vi "Main.vi"() -> ()   [LabVIEW 2013] (continued)
            n812 = call "DB - [Setup].[Item] (Part Details).vi"("DB - Setup Item Enum"=DB_-_Setup_Item_Enum."SELECT [Setup].[ProcedureItem]", "DB.Schema.Table Array"=w1315, "Transaction"=w1292, "DB Refnums"=w1314) -> ("SUMMARY"=w1293:errorcluster)  [unwired: 6 in, 5 out]
            n813 = control-ref of="MCListBox FHS Setup"() -> (w1304:refnum<vi>)
            n814 = local read "WPS Details Setup"() -> (w1310:T8)
            n815 = call "ET3500 - Write Program.vi"("Simulate"=w1309, "Error In"=w1293, "MCListBox FHS Setup"=w1304, "WPS Details Setup"=w1310) -> ("Final Target Temperture"=w1306:i32, "Seq-Seg Info"=w1305:T17)  [unwired: 2 in, 4 out]
            n816 = Number To Decimal String(number=w1306) -> (decimal integer string=w1307:string)  [unwired: 1 in]
            n817 = local write "Seq-Seg Info"(w1305) -> ()
            n818 = Bundle(w1307) -> (w1308:cluster{string})  [unwired: 1 in]
            n819 = local write "Final Target Temperature"(w1308) -> ()
            n820 = Unbundle By Name(w1292) -> ("[TransactionNo]"=w1299:string, "[TransactionRunNo]"=w1303:string)
            n821 = Empty String/Path?(string/path=w1303) -> (empty?=w1298:bool)
            n822 = Select(t="", s=w1298, f=", ") -> (s? t:f=w1302:string)
            n823 = Concatenate Strings(w1299, w1302, w1303) -> (w1297:string)
            n824 = case shown="Error" w1293 {
              tunnel: ["<I 219>" ("<.?....> Message Code") "<E 218>" ("<.?....> Message Code")] -> w1294
              tunnel: ["Transaction Loaded Successfully" ("Short Description (When DB Not Available)") "Transaction Load Fail" ("Short Description (When DB Not Available)")] -> w1295
              tunnel: [" details loaded." ("Description (When DB Not Available)") " cannot be loaded." ("Description (When DB Not Available)")] -> w1296
              frame No Error {
              }
              frame Error {
              }
            }
            n825 = call "Msgbox - Message Handler.vi"("Short Description (When DB Not Available)"=w1295, "Description (When DB Not Available)"=w1296, "Pre-Description"=w1297, "<.?....> Message Code"=w1294) -> ("MHandler Error"=w1291:errorcluster)  [unwired: 5 in, 2 out]
            n826 = local write "MHandler"(w1291) -> ()
          }
          frame True {
            # "Msgbox - Message Handler is already inside"
            # "Event Fired from Search Button"
            n827 = local write "From Search Button"(FALSE ("From Search Button")) -> ()
            n828 = call "DB UI - Search-Load Setup.vi"("Refnums"=w1336) -> ("Error Out"=w1332:errorcluster, "{Cancel}"=w1334:bool, "Transaction"=w1338:T19)  [unwired: 7 in, 1 out]
            n829 = Not(x=w1334) -> (.not. x?=w1333:bool)
            n830 = local write "MHandler"(w1332) -> ()
            n831 = case shown="False" w1333 {
              tunnel: w1338 -> [_ w1341]
              tunnel: [_ w1341] -> w1335
              frame False {
                # "CANCEL is Clicked"
                n832 = call "Queue - EnQueue to MessageQ.vi"("<NoD> Don't Display to UI"=TRUE, "Message"="{Search Setup} Cancelled by user. ") -> ()  [unwired: 9 in, 1 out]
              }
              frame True {
                # "CANCEL NOT Clicked"
                n833 = Unbundle By Name(w1341) -> ("TransactionNo"=w1343:string, "TransactionRunNo"=w1342:string)
                n834 = global write "Global SRTRS.vi" "[TransactionRunNo]"(w1342) -> ()
                n835 = global write "Global SRTRS.vi" "[TransactionNo]"(w1343) -> ()
              }
            }
          }
        }
        n836 = case shown="True" w1250 {
          tunnel: w1253 -> [_ w1290]
          frame False {
          }
          frame True {
            w1271 = string[] ["TC1", "TC2", "TC3", "TC4", "TC5", "TC6"]  # Channel to Probe Cluster Label
            # "Set to NEXT blank value"
            # "Temperature and Time Variant NOT written here."
            # "Do we want to update these values during Load Setup?"
            n837 = control-ref of="Part Details"() -> (w1264:refnum<vi>)
            n838 = control-ref of="WPS Details Setup"() -> (w1263:refnum<vi>)
            n839 = control-ref of="Extra WPS"() -> (w1255:refnum<vi>)
            n840 = property class="Clust (strict)"(reference=w1263) -> ("Value"=w1285:T8)  [unwired: 1 in, 2 out]
            n841 = property class="Str"(reference=w1255) -> ("Value"=w1254:string)  [unwired: 1 in, 2 out]
            n842 = Unbundle By Name(w1290) -> ("TransactionRunNo"=w1268:string)
            n843 = property class="MCListbox (strict)"(reference=w1264) -> (reference out=w1257:refnum<vi>, "ColHdrString"=w1276:string[], "ItemNames"=w1277:string[][])  [unwired: 1 in, 1 out]
            n844 = control-ref of="MCListBox FHS Setup"() -> (w1265:refnum<vi>)
            n845 = local read "Edit WPS in Setup"() -> (w1269:bool)
            n846 = control-ref of="Tab Setup"() -> (w1287:refnum<vi>)
            n847 = control-ref of="No."() -> (w1261:refnum<vi>)
            n848 = Unbundle By Name(w1285) -> ("WPS/Ref"=w1281:T5, "WPS Details Temperature Units"=w1282:string, "Hold Temperature"=w1283:string, "Hold Time (HH:MM)"=w1284:string)
            n849 = Equal?(x=w1268, y="") -> (x = y?=w1266:bool)
            n850 = call "Setup Tab - Enable-Disable.vi"("No."=w1261, "MCListBox FHS Setup"=w1265, "[SRTRS][Config][ParameterSettings] - [userEditableProcedure]"=w1269, "Disabled"=T30."Disabled", "Tab Setup"=w1287) -> ()  [unwired: 7 in]
            n851 = local read "Channel to Probe Mapping"() -> (w1270:cluster{"Channel to Probe Mapping":string})
            n852 = Unbundle By Name(w1270) -> ("Channel to Probe Mapping"=w1272:string)
            n853 = local write "Uploaded to ET"(FALSE ("Uploaded to ET")) -> ()
            n854 = Not(x=w1266) -> (.not. x?=w1259:bool)
            n855 = Array Size(array=w1277) -> (size(s)=w1278:i32[])
            n856 = Index Array(array=w1278) -> (element=w1256:i32)  [unwired: 1 in]
            n857 = property on="TransactionRunNo" class="Str"("Visible"=w1259) -> ()  [unwired: 2 in, 2 out]
            n858 = call "String - Channel to Probe Mappings.vi"("Channel to Probe Mapping"=w1272, "Channel to Probe Cluster Label"=w1271, "ColHdrString"=w1276, "ItemNames"=w1277) -> ("Probe List Valid"=w1274:bool, "Probe List"=w1273:i32[], "cRIO Channel List"=w1275:i32[])  [unwired: 1 in, 4 out]
            n859 = local write "Probe List Valid"(w1274) -> ()
            n860 = local write "Probe List"(w1273) -> ()
            n861 = local write "cRIO Channel List"(w1275) -> ()
            n862 = local write "No. of Items"(w1256) -> ()
            n863 = property on="Transaction Details" class="Bool"("Visible"=w1259) -> ()  [unwired: 2 in, 2 out]
            n864 = local read "Info."() -> (w1279:T9)
            n865 = Bundle By Name(cluster=w1279, "Ref WPS"=w1281, "WPS"=w1254, "Info. Temperature Units"=w1282, "Info. Temperature Units 2"=w1282, "Hold. Temp."=w1283, "Hold. Time (hour:minute)"=w1284) -> (w1280:T9)
            n866 = local write "Info."(w1280) -> ()
            n867 = Increment(x=w1256) -> (x+1=w1258:i32)
            n868 = property class="MCListbox (strict)"(reference=w1257, "Val(Sgnl)"=w1256) -> ()  [unwired: 1 in, 2 out]
            n869 = property on="Setup Edit" class="Bool (strict)"("Value"=FALSE ("Setup Edit")) -> ()  [unwired: 2 in, 2 out]
            n870 = property on="No." class="DigNum (strict)"("Value"=w1258) -> ()  [unwired: 2 in, 2 out]
            n871 = Unbundle By Name(w1290) -> ("TransactionNo"=w1289:string, "TransactionRunNo"=w1288:string)
            n872 = local write "TransactionRunNo (Execute)"(w1288) -> ()
            n873 = local write "Transaction No (Execute)"(w1289) -> ()
            n874 = global write "Global SRTRS.vi" "[TransactionRunNo]"(w1288) -> ()
            n875 = global write "Global SRTRS.vi" "[TransactionNo]"(w1289) -> ()
            n876 = local write "TransactionRunNo"(w1288) -> ()
            n877 = local write "Transaction No"(w1289) -> ()
          }
        }
      }
      event "Transaction Details": Value Change {
        n878 = event-data() -> ()  [unwired: 1 in, 6 out]
        n879 = local read "Transaction No"() -> (w1347:string)
        n880 = local read "TransactionRunNo"() -> (w1346:string)
        n881 = Bundle("Transaction No"=w1347, "TransactionRunNo"=w1346) -> (w1345:T61)  [unwired: 1 in]
        n882 = call "DB UI - Transaction Details.vi"("Transaction"=w1345) -> ("SUMMARY"=w1344:errorcluster)  [unwired: 9 in, 1 out]
        n883 = local write "DB"(w1344) -> ()
      }
      event "SAPProduction Long Text": Value Change {
        n884 = event-data() -> ()  [unwired: 1 in, 6 out]
        n885 = property on="Order No." class="Str"() -> ("Value"=w1350:string)  [unwired: 2 in, 2 out]
        n886 = local read "Logon"() -> (w1349:T21)
        n887 = Unbundle By Name(w1349) -> ("PlantID"=w1348:string)
        n888 = call "DB UI - MasterData SAPProduction Long Text.vi"("[OrderNo]"=w1350, "[PlantId]"=w1348) -> ()  [unwired: 8 in, 2 out]
      }
      event "SAPMaterial Description (Long) Setup Tab", "SAPMaterial Description (Long) Master Data Tab": Value Change {
        n889 = event-data() -> ("CtlRef"=w1353:refnum<vi>)  [unwired: 1 in, 5 out]
        n890 = property class="Bool"(reference=w1353) -> ("Label.Text"=w1352:string)  [unwired: 1 in, 2 out]
        n891 = case shown="\"SAPMaterial Description (Long) Master Data Tab\", Default" w1352 {
          tunnel: [w1357 w1358] -> w1351
          frame "SAPMaterial Description (Long) Master Data Tab", Default {
            n892 = property on="Master Data Material" class="CmbBox"() -> ("Value"=w1357:string)  [unwired: 2 in, 2 out]
          }
          frame "SAPMaterial Description (Long) Setup Tab" {
            n893 = property on="Material" class="CmbBox"() -> ("Value"=w1358:string)  [unwired: 2 in, 2 out]
          }
        }
        n894 = local read "Logon"() -> (w1356:T21)
        n895 = Unbundle By Name(w1356) -> ("LanguageID"=w1355:string)
        n896 = call "DB UI - MasterData SAPMaterial (Long) Description.vi"("FP is Modal"=TRUE ("UI Popup"), "[LanguageId]"=w1355, "[MaterialNo]"=w1351) -> ()  [unwired: 6 in, 3 out]
      }
      event "Read ET3500 Program": Value Change {
        n897 = event-data() -> ()  [unwired: 1 in, 6 out]
        n898 = local read "VISA resource name RS232"() -> (w1362:string)
        n899 = local read "Simulate ET3500"() -> (w1359:bool)
        n900 = call "ET3500 - Read Program.vi"("subVI"=TRUE, "Simulate"=w1359, "VISA resource name"=w1362) -> ("error out"=w1360:errorcluster)  [unwired: 6 in, 2 out]
        n901 = local write "ET3500 Error"(w1360) -> ()
      }
      event "cRIO Set Time": Value Change {
        n902 = event-data() -> ()  [unwired: 1 in, 6 out]
        n903 = call "Password to adjust CompactRIO internal Clock"() -> ("Password"=w1367:string, "OK"=w1368:bool)  [unwired: 17 in, 1 out]
        n904 = case shown="True" w1368 {
          tunnel: w1367 -> [_ w1371]
          tunnel: ["Cancelled.\n" ("message") w1370] -> w1366
          frame False {
          }
          frame True {
            n905 = case shown="\"3504\"" w1371 {
              tunnel: [w1372 "Password OK.\n"] -> w1370
              frame "False", Default {
                w1372 = "Wrong Password.\n" ("message")
                n906 = One Button Dialog(message=w1372) -> ()  [unwired: 1 in, 1 out]
              }
              frame "3504" {
                n907 = local read "Simulate cRIO"() -> (w1375:bool)
                n908 = case shown="False" w1375 {
                  selector: w1375 -> [w1378 _]
                  tunnel: [w1377 _] -> w1373
                  frame False {
                    # "If we are using \"time zone\" string:\nTime Zone strings need to be of the form Etc/GMT-X or Etc/GMT+X where X represents the offset from GMT. For example Etc\\GMT-6 is the equivalent to Central Standard Time in the US. (GMT-5 during Daylight Saving Time). Valid values range from 12 to -13 centered around GMT."
                    n909 = Get Date/Time In Seconds() -> (seconds since 1Jan1904=w1382:timestamp)
                    n910 = case shown="False" FALSE {
                      tunnel: w1382 -> [w1405 w1407]
                      tunnel: [w1405 w1406] -> w1381
                      frame False {
                      }
                      frame True {
                        # "UTC-7 hours"
                        n911 = Multiply(x=60, y=60) -> (x*y=w1410:i32)
                        n912 = Multiply(x=w1410, y=7) -> (x*y=w1408:i32)
                        n913 = Subtract(x=w1407, y=w1408) -> (x-y=w1406:timestamp)
                      }
                    }
                    n914 = local read "cRIO IP"() -> (w1383:string)
                    n915 = call <vilib>:"Initialize Session.vi"("connect timeout in ms (4s)"=u32 5000, "force property refresh (T)"=TRUE, "target (localhost)"=w1383) -> ("error out"=w1387:errorcluster, "session out"=w1388:refnum<k21>)  [unwired: 7 in]
                    n916 = call <vilib>:"Set Time.vi"("error in (no error)"=w1387, "time"=w1381, "session in (localhost)"=w1388) -> ("error out"=w1386:errorcluster, "session out"=w1389:refnum<k21>)  [unwired: 5 in, 2 out]
                    n917 = call-poly <vilib>:"Close.vi"("error in (no error)"=w1386, "session in"=w1389) -> ("error out"=w1379:errorcluster)  [unwired: 9 in]
                    n918 = flat-sequence {
                      tunnel: w1379 -> [w1390]
                      tunnel: w1378 -> [w1398]
                      tunnel: [w1397] -> w1376
                      tunnel: [w1404] -> w1377
                      tunnel: w1376 -> [w1404]
                      frame #0 {
                        n919 = call "Msgbox - Add OR Remove.vi"("Error In"=w1390, "MsgBox"=T44 {"Show"=TRUE, "Priority"=0, "Message"="Setting cRIO Clock...(Done)", "seconds"=1200}) -> ()  [unwired: 8 in, 2 out]
                      }
                      frame #1 {
                        n920 = local read "cRIO Time Sync Tolerance"() -> (w1392:i32)
                        n921 = local read "cRIO shared variable RT Library"() -> (w1396:string)
                        n922 = Concatenate Strings(w1396, "/cRIO Timestamp" ("cRIO Timestamp SV")) -> (w1394:string)
                        n923 = call "cRIO - Check Time Sync.vi"("Time Sync Tolerance (60sec)"=w1392, "Timeout (minutes)"=2, "cRIO Timestamp SV"=w1394) -> ("error out 4"=w1399:errorcluster)  [unwired: 5 in, 3 out]
                        n924 = local read "cRIO Data Retention"() -> (w1402:i32)
                        n925 = control-ref of="cRIO Status"() -> (w1400:refnum<vi>)
                        n926 = call "cRIO - Shared Variable RW.vi"("shared variable RT Library"=w1396, "Read/Write"=cRIO_RW_Enum."Write Others", "Error In"=w1399, "Simulate cRIO"=w1398, "cRIO Data Retention"=w1402, "cRIO Status"=w1400) -> ("Error Out"=w1397:errorcluster)  [unwired: 5 in, 8 out]
                      }
                      frame #2 {
                        n927 = call "Msgbox - Add OR Remove.vi"("MsgBox"=T44 {"Show"=FALSE, "Priority"=0, "Message"="Setting cRIO Clock...(Done)", "seconds"=1200}) -> ()  [unwired: 9 in, 2 out]
                      }
                    }
                  }
                  frame True {
                    n928 = One Button Dialog(message="cRIO Simulate Set Time OK.") -> ()  [unwired: 1 in, 1 out]
                  }
                }
                n929 = local write "cRIO Error"(w1373) -> ()
              }
            }
          }
        }
        n930 = Concatenate Strings("[cRIO Set Time] Clicked by User. " ("element"), w1366) -> (w1364:string)
        n931 = call "Queue - EnQueue to MessageQ.vi"("<NoD> Don't Display to UI"=TRUE, "Message"=w1364) -> ()  [unwired: 9 in, 1 out]
      }
      event Mouse Down? {
        n932 = event-data() -> ()  [unwired: 1 in, 8 out]
        n933 = local read "DB - Master Data Load"() -> (w1414:bool)
        n934 = case shown="True" w1414 {
          frame False {
          }
          frame True {
            n935 = global read "Global SRTRS.vi" "Logon"() -> (w1419:T21)
            n936 = Unbundle By Name(w1419) -> ("PlantID"=w1418:string)
            n937 = call "DB - [MasterData].[OutputSet].vi"("[PlantId]"=w1418) -> ("2D data"=w1417:string[][])  [unwired: 6 in, 4 out]
            "[OutputSetId],[Description]" <- w1417
            n938 = Index Array(array=w1417, index (col)=0 ("disabled index (col)")) -> (element=w1415:string[])  [unwired: 1 in]
            n939 = property on="Output Set" class="CmbBox (strict)"("Strings[]"=w1415) -> ()  [unwired: 2 in, 2 out]
          }
        }
        n940 = event-data() -> ()  [unwired: 2 in, 1 out]
      }
      event Value Change {
        # "Set [Description] based on [OutputSetId] Chosen"
        # "Set [Description] based on [OutputSetId] Chosen"
        n941 = event-data() -> ("NewVal"=w1424:T5)  [unwired: 1 in, 5 out]
        n942 = local read "[OutputSetId],[Description]"() -> (w1427:string[][])
        n943 = Index Array(array=w1427, index (col) #1=0 ("disabled index (col)"), index (col) #2=1 ("index (col)")) -> (element #1=w1425:string[], element #2=w1421:string[])  [unwired: 2 in]
        n944 = Search 1D Array(1D array=w1425, element=w1424) -> (index of element=w1423:i32)  [unwired: 1 in]
        n945 = Index Array(array=w1421, index=w1423) -> (element=w1420:string)
        n946 = property on="Description" class="Str"("Value"=w1420) -> ()  [unwired: 2 in, 2 out]
      }
      event "Setup Load Debug": Value Change {
        w1455 = string[] ["TC1", "TC2", "TC3", "TC4", "TC5", "TC6"]  # Channel to Probe Cluster Label
        # "We are using CellBG Unused Cells color for both\nMCListBox FHS Setup\nMCListBox AWPS"
        # "Part Details\nMCListBox FHS Setup\nMCListBox AWPS"
        # "Only WPS Detais Setup"
        # "MCListBox FHS Setup\nMCListBox AWPS"
        # "For Debug ONLY"
        n947 = event-data() -> ()  [unwired: 1 in, 6 out]
        n948 = control-ref of="WPS Details Setup"() -> (w1438:refnum<vi>)
        n949 = Index Array(array=w1463, index #1=0 ("index"), index #2=1 ("index"), index #3=2 ("index")) -> (element #1=w1450:refnum<vi>, element #2=w1462:refnum<vi>, element #3=w1461:refnum<vi>)
        n950 = local read "Setup"() -> (w1434:path)
        n951 = Build Array(w1450, w1462, w1461) -> (w1460:refnum<vi>[])
        n952 = Format Date/Time String(time format string (%c)="%Y\\%m") -> (date/time string=w1433:string)  [unwired: 2 in]
        n953 = Build Array "Part Details\nClusters"(w1438) -> (w1464:refnum<vi>[])
        n954 = local read "Channel to Probe Mapping"() -> (w1456:cluster{"Channel to Probe Mapping":string})
        n955 = Unbundle By Name(w1456) -> ("Channel to Probe Mapping"=w1454:string)
        n956 = Build Path(base path=w1434, name or relative path=w1433) -> (appended path=w1432:path)
        n957 = call "File Dialog"("start path"=w1432, "prompt"="Select SETUP file", "pattern (all files)"="*.stp" ("pattern label")) -> ("selected path"=w1476:path, "error out"=w1480:errorcluster)  [unwired: 9 in, 2 out]
        n958 = call <vilib>:"Open Config Data.vi"("error in (no error)"=w1480, "configuration file path"=w1476) -> ("error out"=w1479:errorcluster, "refnum"=w1481:T59)  [unwired: 7 in, 1 out]
        n959 = Strip Path(path=w1476) -> (name=w1475:string)  [unwired: 1 out]
        n960 = for {
          tunnel: w1460 -> [w1495] mode=indexing
          tunnel: w1481 -> [w1499]
          tunnel: w1479 -> [w1498]
          tunnel: [w1497] -> w1478
          tunnel: [w1496] -> w1477
          n961 = call "Key - MCListbox Read.vi"("error in (no error)"=w1498, "New MulticolumnListbox Ref"=w1495, "Original MulticolumnListbox Ref"=w1495, "refnum"=w1499) -> ("error out"=w1496:errorcluster, "Refnum out"=w1497:T59)  [unwired: 4 in, 2 out]
        }
        n962 = Match Pattern(string=w1475, regular expression="[_]") -> (before substring=w1430:string)  [unwired: 1 in, 3 out]
        n963 = global write "Global SRTRS.vi" "[TransactionNo]"(w1430) -> ()
        n964 = local write "Transaction No (Execute)"(w1430) -> ()
        n965 = local write "Transaction No"(w1430) -> ()
        n966 = for {
          tunnel: w1464 -> [w1490] mode=indexing
          tunnel: w1478 -> [w1494]
          tunnel: w1477 -> [w1493]
          tunnel: [w1492] -> w1470
          tunnel: [w1491] -> w1471
          n967 = call "Key - Cluster Read.vi"("error in (no error)"=w1493, "New Ctl Ref"=w1490, "Original Ctl Ref"=w1490, "Refnum in"=w1494) -> ("error out"=w1492:errorcluster, "Refnum out"=w1491:T59)  [unwired: 5 in, 1 out]
        }
        n968 = call <vilib>:"Close Config Data.vi"("error in (no error)"=w1470, "refnum"=w1471) -> ("error out"=w1448:errorcluster, "file path"=w1482:path)  [unwired: 8 in]
        n969 = property class="MCListbox (strict)"(reference=w1450, error in=w1448) -> (error out=w1436:errorcluster, "ColHdrString"=w1449:string[], "ItemNames"=w1441:string[][])  [unwired: 1 out]
        n970 = property class="Clust (strict)"(reference=w1438, error in=w1436) -> (error out=→"Property Node Error":errorcluster, "Value"=w1437:T8)  [unwired: 1 out]
        n971 = Array Size(array=w1441) -> (size(s)=w1440:i32[])
        n972 = Unbundle By Name(w1437) -> ("WPS/Ref"=w1445:T5, "WPS Details Temperature Units"=w1444:string, "Hold Temperature"=w1443:string, "Hold Time (HH:MM)"=w1442:string)
        n973 = Index Array(array=w1440) -> (element=w1439:i32)  [unwired: 1 in]
        n974 = call "String - Channel to Probe Mappings.vi"("Channel to Probe Mapping"=w1454, "Channel to Probe Cluster Label"=w1455, "ColHdrString"=w1449, "ItemNames"=w1441) -> ("Probe List Valid"=w1452:bool, "Probe List"=w1453:i32[], "cRIO Channel List"=w1451:i32[])  [unwired: 1 in, 4 out]
        n975 = local write "Probe List Valid"(w1452) -> ()
        n976 = local write "Probe List"(w1453) -> ()
        n977 = local write "cRIO Channel List"(w1451) -> ()
        n978 = local write "No. of Items"(w1439) -> ()
        n979 = Index Array(array=w1463, index #1=1 ("index"), index #2=2 ("index")) -> (element #1=w1467:refnum<vi>, element #2=w1466:refnum<vi>)
        n980 = Build Array(w1467, w1466) -> (w1465:refnum<vi>[])
        n981 = local read "Info."() -> (w1447:T9)
        n982 = Bundle By Name(cluster=w1447, "Ref WPS"=w1445, "Info. Temperature Units"=w1444, "Info. Temperature Units 2"=w1444, "Hold. Temp."=w1443, "Hold. Time (hour:minute)"=w1442) -> (w1446:T9)
        n983 = local write "Info."(w1446) -> ()
        n984 = Not A Number/Path/Refnum?(number/path/refnum=w1482) -> (NaN/Path/Refnum?=w1483:bool)
        n985 = for {
          tunnel: w1465 -> [w1489] mode=indexing
          tunnel: w1448 -> [w1488]
          n986 = local read "CellBG Unused Cells"() -> (w1485:u32)
          n987 = call "MCListbox Refresh.vi"("Which Cells"=T46."Exisiting and Blank Cells", "Error In"=w1488, "color of New Cells"=w1485, "color of Blank cells"=w1485, "MulticolumnListbox in"=w1489) -> ("Error Out"=w1486:errorcluster)  [unwired: 5 in, 1 out]
          n988 = local write "Property Node Error"(w1486) -> ()
        }
        n989 = case "MessageQ" shown="False" w1483 {
          tunnel: w1482 -> [w1506 _]
          tunnel: [w1503 w1507] -> w1429
          tunnel: "{Load Setup}" ("result string") -> [w1501 w1509]
          frame False {
            w1504 = "\"" ("string")
            # "File Load OK"
            n990 = Path To String(path=w1506) -> (string=w1505:string)
            n991 = Concatenate Strings(w1501, " OK. " ("string"), w1504, w1505, w1504, " loaded." ("string")) -> (w1503:string)
          }
          frame True {
            # "File Not Loaded"
            n992 = Concatenate Strings(w1509, " Cancelled.") -> (w1507:string)
          }
        }
        n993 = call "Queue - EnQueue to MessageQ.vi"("<NoD> Don't Display to UI"=TRUE, "Message"=w1429) -> ()  [unwired: 9 in, 1 out]
      }
      event "------------------------------------        Execute TAB      ------------------------------------": Value Change {
        n994 = event-data() -> ()  [unwired: 1 in, 6 out]
      }
      event "Recipe Stop", "Recipe Start": Value Change {
        w1511 = 1  # MCListBox FHS Setup
        # "[BUTTON ACTIONS] are logged into MessageQ"
        n995 = event-data() -> ()  [unwired: 1 in, 6 out]
        n996 = Index Array(array=w1512, index=w1511) -> (element=w1510:refnum<vi>)
        n997 = case shown="True" "Recipe Stop" {
          frame False {
          }
          frame True {
            # "User Click STOP"
            n998 = call "Msgbox - Message Handler.vi"("Short Description (When DB Not Available)"="Process Stop", "Description (When DB Not Available)"="Data Logging in progress. Do you want process to stop?", "<.?....> Message Code"="<W 307>") -> ("MHandler Error"=w1651:errorcluster, "OK Out"=w1650:bool)  [unwired: 6 in, 1 out]
            "Manual Stop" <- w1650
            n999 = local write "MHandler"(w1651) -> ()
            n1000 = local write "Recipe Stop Flag"(w1650) -> ()
            n1001 = Select(t="OK." ("Message"), s=w1650, f="Cancel." ("Message")) -> (s? t:f=w1653:string)
            n1002 = Concatenate Strings("{Recipe Stop} User clicks " ("string"), w1653) -> (w1660:string)
            n1003 = call "Queue - EnQueue to MessageQ.vi"("<NoD> Don't Display to UI"=TRUE, "Message"=w1660) -> ()  [unwired: 9 in, 1 out]
          }
        }
        n1004 = case shown="True" "Recipe Start" {
          selector: "Recipe Start" -> [w1516 _]
          tunnel: [w1516 w1518] -> w1513
          tunnel: w1510 -> [_ w1517]
          frame False {
            (unwired) ""
          }
          frame True {
            n1005 = local read "Uploaded to ET"() -> (w1519:bool)
            n1006 = case shown="False" w1519 {
              selector: w1519 -> [_ w1649]
              tunnel: [w1520 w1649] -> w1518
              tunnel: w1517 -> [w1523 _]
              frame False {
                # "Current [TransactionNo] (and) [TransactionRunNo] may not be the last one UPLOADED to ET. Must UPLOAD again."
                n1007 = local read "VISA resource name RS232"() -> (w1526:string)
                n1008 = local read "WPS Details Setup"() -> (w1527:T8)
                n1009 = local read "Simulate ET3500"() -> (w1525:bool)
                n1010 = call "ET3500 - Write Program.vi"("Simulate"=w1525, "MCListBox FHS Setup"=w1523, "WPS Details Setup"=w1527, "VISA resource name RS232"=w1526) -> ("ET3500"=w1521:errorcluster, "Final Target Temperture"=w1524:i32, "Seq-Seg Info"=w1522:T17)  [unwired: 2 in, 3 out]
                n1011 = local write "Seq-Seg Info"(w1522) -> ()
                n1012 = flat-sequence {
                  tunnel: w1524 -> [w1530]
                  frame #0 {
                    n1013 = Number To Decimal String(number=w1530) -> (decimal integer string=w1529:string)  [unwired: 1 in]
                    n1014 = Bundle(w1529) -> (w1528:cluster{string})  [unwired: 1 in]
                    n1015 = property on="Final Target Temperature" class="Clust (strict)"("Value"=w1528) -> ()  [unwired: 2 in, 2 out]
                  }
                }
                n1016 = local write "ET3500 Error"(w1521) -> ()
                n1017 = case shown="No Error" w1521 {
                  tunnel: w1525 -> [w1532 _]
                  tunnel: [w1531 FALSE] -> w1520
                  frame No Error {
                    n1018 = while {
                      tunnel: w1532 -> [w1536]
                      tunnel: [w1533] -> w1531
                      i -> [w1535]
                      stop <- w1534 stop-if-true
                      n1019 = case shown="2, Default" w1535 {
                        tunnel: w1536 -> [_ _ w1618]
                        tunnel: [w1548 TRUE w1614] -> w1534
                        tunnel: [w1548 FALSE ("OK Out") w1613] -> w1533
                        frame 1 {
                          w1546 = 7  # Cal. Required
                          (unwired) string[] ["Name", "Model", "Serial No.", "Last Cal. Date", "Next Cal. Due Date", "Equipment ID", "Notice Period", "Cal. Required"]  # 2015-01-01 11:16 ColHdr[]
                          w1556 = 5  # Equipment ID
                          w1562 = 6  # Notice Period
                          w1564 = 4  # Next Cal. Due Date
                          # "Temperature Controller follows Furnace date"
                          # "Equipment ID Notice Due List"
                          # "Not Prompted here. Only in Setup"
                          # "If ALL TRUE End Loop, SET\nUploaded to ET to TRUE"
                          # "Same Check done in {Setup Save}"
                          # "60 x 60 x 24 = 86,400 seconds/day"
                          # "2nd Check: Are Equipment Calibration OK?"
                          n1020 = property on="Equipment Details" class="MCListbox (strict)"() -> ("ItemNames"=w1555:string[][])  [unwired: 2 in, 2 out]
                          n1021 = property on="Next Calibration Due Date" class="Str"() -> ("Value"=w1563:string)  [unwired: 2 in, 2 out]
                          n1022 = Array Size(array=w1555) -> (size(s)=w1554:i32[])
                          n1023 = Index Array(array=w1554) -> (element=w1553:i32)  [unwired: 1 in]
                          n1024 = Index Array(array=w1555, index (col) #1=w1564, index (col) #2=w1562, index (col) #3=w1556, index (col) #4=w1546) -> (element #1=w1537:string[], element #2=w1538:string[], element #3=w1543:string[], element #4=w1545:string[])  [unwired: 4 in]
                          n1025 = Greater Than 0?(x=w1553) -> (x > 0?=w1549:bool)
                          n1026 = local write "Equipment Details Complete"(w1549) -> ()
                          n1027 = Build Array (concatenate)(w1563, w1537) -> ()  [unwired: 1 out]
                          n1028 = call "DB - Convert BIT Type.vi"("BIT Type (eg Inactive) (Array)"=w1545) -> ("Boolean (Array)"=w1542:bool[])  [unwired: 2 in, 2 out]
                          n1029 = Get Date/Time In Seconds() -> (seconds since 1Jan1904=w1544:timestamp)
                          n1030 = property on="Output Set" class="CmbBox (strict)"() -> ("Value"=w1552:T5)  [unwired: 2 in, 2 out]
                          n1031 = Empty String/Path?(string/path=w1552) -> (empty?=w1551:bool)
                          n1032 = local read "Date Format (UserDefined)"() -> (w1541:string)
                          n1033 = for {
                            tunnel: w1537 -> [w1579] mode=indexing
                            tunnel: w1544 -> [w1569]
                            tunnel: [w1573] -> w1539 mode=indexing
                            tunnel: w1538 -> [w1583] mode=indexing
                            tunnel: w1543 -> [w1572] mode=indexing
                            tunnel: [w1572] -> _ mode=indexing if=w1580
                            tunnel: w1541 -> [w1578]
                            tunnel: w1542 -> [w1577] mode=indexing
                            tunnel: [w1572] -> w1540 mode=indexing if=w1571
                            # "All FALSE will\nCreate DUE list"
                            # "Next Cal Due Date - Today\n<= Notice Period"
                            n1034 = Not(x=w1577) -> (.not. x?=w1575:bool)
                            n1035 = call "String - Convert UserDefined Date to SQL Date (YYYY-mm-dd).vi"("Date Format (UserDefined)"=w1578, "Date String (UserDefined)"=w1579) -> ("time stamp"=w1570:timestamp)  [unwired: 7 in, 2 out]
                            n1036 = Decimal String To Number(string=w1583) -> (number=w1581:i32)  [unwired: 2 in, 1 out]
                            n1037 = Greater?(x=w1570, y=w1569) -> (0:w1576:bool)
                            n1038 = Or(x=w1576, y=w1575) -> (x .or. y?=w1573:bool)
                            n1039 = Multiply(x=86400.0, y=w1581) -> (x*y=w1567:dbl)
                            n1040 = Subtract(x=w1570, y=w1569) -> (x-y=w1568:dbl)
                            n1041 = Less Or Equal?(x=w1568, y=w1567) -> (x <= y?=w1566:bool)
                            n1042 = Compound Arithmetic op=OR "OR"(invert w1573, invert w1566, w1575) -> (w1574:bool)
                            n1043 = Not(x=w1574) -> (.not. x?=w1580:bool)
                            n1044 = Not(x=w1573) -> (.not. x?=w1571:bool)
                          }
                          n1045 = Not(x=w1551) -> (.not. x?=w1547:bool)
                          n1046 = local write "Output Set Details Complete"(w1547) -> ()
                          n1047 = Array To Spreadsheet String(delimiter (Tab)=",", array=w1540, 3:"" ("format string")) -> (spreadsheet string=w1558:string)
                          n1048 = local write "Calibration Date OK"(w1539) -> ()
                          n1049 = And Array Elements(Boolean array=w1539) -> (logical AND=w1550:bool)
                          n1050 = Search and Replace String(replace all?=TRUE ("replace all? (F)"), input string=w1558, search string="\r\n") -> (result string=w1565:string)  [unwired: 5 in, 3 out]
                          n1051 = local write "All Calibration Date Valid"(w1550) -> ()
                          n1052 = local write "Equipment ID Due List"(w1565) -> ()
                          n1053 = Compound Arithmetic op=AND(w1550, w1549, w1547) -> (w1548:bool)
                        }
                        frame 2, Default {
                          # "One of these is FALSE"
                          # "Prompt Errors of 2nd Check...if any"
                          n1054 = local read "Equipment Details Complete"() -> (w1586:bool)
                          n1055 = local read "Output Set Details Complete"() -> (w1585:bool)
                          n1056 = local read "All Calibration Date Valid"() -> (w1587:bool)
                          n1057 = case shown="True" w1587 {
                            tunnel: ["<E 213>" w1602] -> w1590
                            tunnel: [" calibration validity expired. Save Cancelled." w1601] -> w1591
                            tunnel: ["Calibration Expired" w1600] -> w1592
                            tunnel: [w1595 _] -> w1589
                            tunnel: w1586 -> [_ w1599]
                            tunnel: w1585 -> [_ w1598]
                            frame False {
                              # "Calibration Expired"
                              n1058 = local read "Equipment ID Due List"() -> (w1595:string)
                            }
                            frame True {
                              # "All Calibration Date Valid"
                              n1059 = case shown="True" w1599 {
                                tunnel: ["<E 214>" w1606] -> w1602
                                tunnel: ["Save Cancelled." w1608] -> w1601
                                tunnel: ["Equipment Not Available. " w1607] -> w1600
                                tunnel: w1598 -> [_ w1609]
                                frame False {
                                # "Equipment Not Available"
                                }
                                frame True {
                                # "Equipment Details Complete"
                                n1060 = case shown="False" w1609 {
                                tunnel: ["Please select a valid Output Set to proceed" _] -> w1608
                                tunnel: ["Output Set Not Assigned" _] -> w1607
                                tunnel: ["<E 215>" _] -> w1606
                                frame False {
                                # "Output Set Details Incomplete"
                                }
                                frame True {
                                # "NA becasue all conditions \nare ANDed\nSo at least one would have failed"
                                # "Output Set Details Complete"
                                }
                                }
                                }
                              }
                            }
                          }
                          n1061 = call "Msgbox - Message Handler.vi"("Short Description (When DB Not Available)"=w1592, "Description (When DB Not Available)"=w1591, "Pre-Description"=w1589, "<.?....> Message Code"=w1590) -> ("MHandler Error"=w1588:errorcluster)  [unwired: 5 in, 2 out]
                          n1062 = local write "MHandler"(w1588) -> ()
                        }
                        frame 0 {
                          # "1st Check: Variants Valid?"
                          n1063 = property on="Variant Allowed (Hold Time)" class="DigNum (strict)"() -> ("Value"=w1622:dbl)  [unwired: 2 in, 2 out]
                          n1064 = property on="Variant Allowed (Hold Temp)" class="DigNum (strict)"() -> ("Value"=w1623:dbl)  [unwired: 2 in, 2 out]
                          n1065 = Equal To 0?(x=w1623) -> (x = 0?=w1621:bool)
                          n1066 = Equal To 0?(x=w1622) -> (x = 0?=w1620:bool)
                          n1067 = Or(x=w1621, y=w1620) -> (x .or. y?=w1619:bool)
                          n1068 = case shown="True" w1619 {
                            tunnel: [TRUE ("OK Out") w1635] -> w1613
                            tunnel: ["" w1630] -> w1617
                            frame False {
                            }
                            frame True {
                              # "Either one is ZERO"
                              n1069 = call "Msgbox - Message Handler.vi"("Short Description (When DB Not Available)"="Temperature/Time Allowance Not Set", "Description (When DB Not Available)"="Variance allowed for Hold. Temperature and Holding Time is not set. Do you want to proceed?", "<.?....> Message Code"="<W 302>") -> ("MHandler Error"=w1637:errorcluster, "OK Out"=w1635:bool)  [unwired: 6 in, 1 out]
                              n1070 = local write "MHandler"(w1637) -> ()
                              n1071 = Select(t="OK.", s=w1635, f="Cancel.") -> (s? t:f=w1631:string)
                              n1072 = Concatenate Strings("User Select ", w1631) -> (w1630:string)
                            }
                          }
                          n1073 = Select(t="Simulate Upload to ET3504 OK." ("message"), s=w1618, f="Upload to ET3504 OK." ("message")) -> (s? t:f=w1624:string)
                          n1074 = Concatenate Strings("{Recipe Start} " ("string"), w1624, w1617) -> (w1615:string)
                          n1075 = call "Queue - EnQueue to MessageQ.vi"("<NoD> Don't Display to UI"=TRUE, "Message"=w1615) -> ()  [unwired: 9 in, 1 out]
                          n1076 = Not(x=w1613) -> (.not. x?=w1614:bool)
                        }
                      }
                    }
                  }
                  frame Error {
                    n1077 = call "Msgbox - Message Handler.vi"("Short Description (When DB Not Available)"="Heating Sequence Upload Fail", "Description (When DB Not Available)"="Heating sequence program upload to furnace controller fail. Check the controller and retry", "<.?....> Message Code"="<E 220>") -> ("MHandler Error"=w1644:errorcluster)  [unwired: 6 in, 2 out]
                    n1078 = local write "MHandler"(w1644) -> ()
                    n1079 = call "Queue - EnQueue to MessageQ.vi"("<NoD> Don't Display to UI"=TRUE, "Message"="{Recipe Start} Upload to ET3504 Failed. Check if ET3504 is already Running a Program. Check communication cable to ET3504." ("message")) -> ()  [unwired: 9 in, 1 out]
                  }
                }
                n1080 = local write "Uploaded to ET"(w1520) -> ()
              }
              frame True {
                # "Already Uploaded, can START"
                n1081 = call "Queue - EnQueue to MessageQ.vi"("<NoD> Don't Display to UI"=TRUE, "Message"="{Recipe Start} ET3504 already uploaded by a previous same TransactionNo." ("string")) -> ()  [unwired: 9 in, 1 out]
              }
            }
          }
        }
        n1082 = local write "Recipe Start Flag"(w1513) -> ()
      }
      event "Parameter": Value Change {
        n1083 = event-data() -> ()  [unwired: 1 in, 6 out]
        n1084 = local read "DB - Transaction"() -> (w1664:bool)
        n1085 = case shown="True" w1664 {
          tunnel: [w1665 w1680] -> w1663
          frame False {
            n1086 = local read "Latest stp file"() -> (w1668:path)
            n1087 = control-ref of="Parameter Buffer"() -> (w1672:refnum<vi>)
            n1088 = call <vilib>:"Open Config Data.vi"("create file if necessary (T)"=FALSE, "configuration file path"=w1668) -> ("error out"=w1666:errorcluster, "refnum"=w1669:T59)  [unwired: 7 in, 1 out]
            n1089 = call "Key - Cluster Read.vi"("error in (no error)"=w1666, "New Ctl Ref"=w1672, "Original Ctl Ref"=w1672, "Refnum in"=w1669) -> ("error out"=w1667:errorcluster, "Refnum out"=w1671:T59)  [unwired: 5 in, 1 out]
            n1090 = call <vilib>:"Close Config Data.vi"("error in (no error)"=w1667, "write file if changed (T)"=FALSE, "refnum"=w1671) -> ("error out"=w1665:errorcluster)  [unwired: 7 in, 1 out]
          }
          frame True {
            w1683 = T62[] [enum."[StartHoldTime]", enum."[EndHoldTime]", enum."[StartHoldTemp]", enum."[EndHoldTemp]"] items=["[StartRecordTime]", "[StartRecordTemp]", "[MaxRecordedTemp]", "[MaxRecordedTempTime]", "[MinRecordedTemp]", "[MinRecordedTempTime]", "[EndRecordTemp]", "[EndRecordTime]", "[RecordedMinutes]", "[StartHoldTime]", "[StartHoldTemp]", "[HoldTimeMaxTemp]", "[HoldTimeMaxTempTime]", "[HoldTimeMinTemp]", "[HoldTimeMinTempTime]", "[EndHoldTime]", "[EndHoldTemp]", "[HoldDurationMinutes]", "[TempDiffDuringHold]", "[UnitOfTemperature]", "[PerformedBy]", "[PerformedOn]", "[IsTempWithinTol]", "[IsTimeWithinTol]", "[HoldTimePercentage]", "[ProcessStatus]", "[OverallStatus]", "[SequenceStatus]", "[Parameter1]", "[Parameter2]", "[Parameter3]", "[Parameter4]", "[Parameter5]", "[Parameter6]", "[Parameter7]", "[Parameter8]", "[Parameter9]", "[Parameter10]", "[Parameter11]", "[Parameter12]", "[Result]", "[RawDataFile]", "[RawDataFilePath]", "[RawDataFileName]", "[OutputSetId]", "[SavedBy]", "[SavedOn]", "[Inactive]"] ("[TransactionResult] v02")
            n1091 = local read "TransactionRunNo"() -> (w1685:string)
            n1092 = local read "Transaction No"() -> (w1686:string)
            n1093 = Bundle("Transaction No"=w1686, "TransactionRunNo"=w1685) -> (w1684:T61)  [unwired: 1 in]
            n1094 = call "DB - [Execute].[Transaction].vi"("DB.Schema.Table"="SRTRS.Execute.TransactionResult", "Transaction"=w1684, "DB - Execute Transaction"=DB_-_Execute_Transaction_Enum."SELECT [TransactionResult]", "[TransactionResult] v02"=w1683) -> ("1D Results"=w1674:string[], "SUMMARY"=w1680:errorcluster)  [unwired: 12 in, 2 out]
            n1095 = Index Array(array=w1674, index #1=0 ("index")) -> (element #1=w1679:string, element #2=w1678:string, element #3=w1677:string, element #4=w1676:string)  [unwired: 3 in]
            n1096 = local read "Parameter Buffer"() -> (w1682:T15)
            n1097 = Bundle By Name(cluster=w1682, "Start Holding Time and Date"=w1679, "End Holding Time and Date"=w1678, "Start Holding Temperature"=w1677, "End Holding Temperature"=w1676) -> (w1681:T15)
            n1098 = local write "Parameter Buffer"(w1681) -> ()
          }
        }
        n1099 = case shown="No Error" w1663 {
          frame No Error {
            n1100 = local read "Parameter Buffer"() -> (w1710:T15)
            n1101 = Unbundle By Name(w1710) -> ("Start Holding Time and Date"=w1704:string, "End Holding Time and Date"=w1702:string, "Start Holding Temperature"=w1709:string, "End Holding Temperature"=w1708:string)
            n1102 = property on="Part Details" class="MCListbox (strict)"() -> ("ItemNames"=w1698:string[][])  [unwired: 2 in, 2 out]
            n1103 = for {
              tunnel: w1698 -> [w1714] mode=indexing
              tunnel: [w1712] -> w1697 mode=indexing
              w1713 = 1  # Order No
              n1104 = Index Array(array=w1714, index=w1713) -> (element=w1712:string)
            }
            n1105 = Fract/Exp String To Number(string=w1709) -> (number=w1707:dbl)  [unwired: 3 in, 1 out]
            n1106 = Fract/Exp String To Number(string=w1708) -> (number=w1706:dbl)  [unwired: 3 in, 1 out]
            n1107 = call "String - Convert Str (YYYY-mm-dd HHcMMcSS) to TimeStamp.vi"("YYYY-mm-dd HH:MM:SS (String)"=w1704) -> ("time stamp"=w1703:timestamp)  [unwired: 9 in, 1 out]
            n1108 = call "String - Convert Str (YYYY-mm-dd HHcMMcSS) to TimeStamp.vi"("YYYY-mm-dd HH:MM:SS (String)"=w1702) -> ("time stamp"=w1701:timestamp)  [unwired: 9 in, 1 out]
            n1109 = property on="Variant Allowed (Hold Temp)" class="Bool (strict)"() -> ("Value"=w1705:bool)  [unwired: 2 in, 2 out]
            n1110 = Array To Spreadsheet String(delimiter (Tab)=",", array=w1697, 3:"" ("format string")) -> (spreadsheet string=w1692:string)
            n1111 = local read "Info."() -> (w1711:T9)
            n1112 = Search and Replace String(replace all?=TRUE ("replace all? (F)"), input string=w1692, search string="\r\n") -> (result string=w1691:string)  [unwired: 5 in, 3 out]
            n1113 = call "Parameters - Update.vi"("Parameter (End Dwell Temp)"=w1706, "Variant Allowed (Summarised)"=w1705, "Parameter (Start Dwell Temp)"=w1707, "Parameter (End Dwell Time)"=w1701, "Parameter (Start Dwell Time)"=w1703, "Info."=w1711) -> ("Parameters"=w1700:string[][])  [unwired: 2 in, 3 out]
            n1114 = Build Array("Order(s)" ("element"), w1691) -> (w1693:string[])
            n1115 = Build Array (concatenate)(w1693, w1700) -> (w1699:string[][])
            n1116 = call "Parameters UI - Dialog Box.vi"("Parameters"=w1699) -> ()  [unwired: 10 in]
          }
          frame Error {
          }
        }
        n1117 = call "Queue - EnQueue to MessageQ.vi"("<NoD> Don't Display to UI"=TRUE, "Message"="{Key Parameters} Clicked By User." ("string")) -> ()  [unwired: 9 in, 1 out]
      }
      event "Toggle ET3500 Error": Value Change {
        w1721 = T63[] [enum."[Message1]"] items=["[IsActive]", "[TransactionNo]", "[TransactionRunNo]", "[SequenceStatus]", "[StartRecordTime]", "[EndRecordTime]", "[StartHoldTime]", "[EndHoldTime]", "[Message1]", "[Message2]", "[HoldTimeRemaining]", "[HoldTimePercentage]", "[HoldProgressColor]", "[OrderNumbers]", "[CurrentTemp]", "[UnitOfTemperature]", "[IsAppClientLive]", "[RawDataFile]", "[RecordedMinutes]", "[FurnaceControlStatus]", "[FurnaceControlColor]", "[ControllerStatus]", "[ControllerColor]", "[IsControllerOnline]", "[ProcessColor]", "[OverallColor]", "[LastUpdatedOn]", "[LastUpdatedCmsTime]", "[Inactive]"] ("[Execute].[ActiveProcess]\n2014-10-14 14:58")
        n1118 = event-data() -> ("NewVal"=w1727:string)  [unwired: 1 in, 5 out]
        n1119 = case shown="\"<E 306>\", Default" w1727 {
          selector: w1727 -> [w1733 w1741]
          tunnel: [w1734 w1745] -> w1730
          tunnel: ["Hold. Time Exceed Fail" ("Short Description (When DB Not Available)") "Hold. Temperature Fail" ("Short Description (When DB Not Available)")] -> w1719
          tunnel: [" is the current hold. Duration. But the hold. time and variance allowed are respectively: " ("Short Description (When DB Not Available)") " is the current temperature. But the hold. temperature and variance allowed are respectively: " ("Short Description (When DB Not Available)")] -> w1729
          tunnel: [w1732 w1742] -> w1728
          tunnel: [w1733 w1741] -> w1726
          frame "<E 306>", Default {
            n1120 = local read "<current hold time> ON Failing Hold Time Variance"() -> (w1732:string)
            n1121 = property on="Variant Allowed (Hold Time)" class="DigNum (strict)"() -> ("Value"=w1737:dbl)  [unwired: 2 in, 2 out]
            n1122 = property on="Hold. Time (hour:minute)" class="Str"() -> ("Value"=w1731:string)  [unwired: 2 in, 2 out]
            n1123 = Number To Fractional String(number=w1737, precision (6)=i16 0) -> (F-format string=w1735:string)  [unwired: 2 in]
            n1124 = Concatenate Strings(w1731, ", " ("string"), w1735) -> (w1734:string)
          }
          frame "<E 305>" {
            n1125 = local read "<current temperature> ON Failing Hold Temp Variance"() -> (w1742:string)
            n1126 = property on="Variant Allowed (Hold Temp)" class="DigNum (strict)"() -> ("Value"=w1750:dbl)  [unwired: 2 in, 2 out]
            n1127 = property on="Hold. Temp." class="Str"() -> ("Value"=w1749:string)  [unwired: 2 in, 2 out]
            n1128 = property on="Info. Temperature Units" class="Str"() -> ("Value"=w1746:string)  [unwired: 2 in, 2 out]
            n1129 = Number To Fractional String(number=w1750, precision (6)=i16 0) -> (F-format string=w1747:string)  [unwired: 2 in]
            n1130 = Concatenate Strings(w1749, w1746, ", " ("string"), w1747, w1746) -> (w1745:string)
          }
        }
        n1131 = local read "Logon"() -> (w1718:T21)
        n1132 = call "Msgbox - Message Handler.vi"("Short Description (When DB Not Available)"=w1719, "Description (When DB Not Available)"=w1729, "Post-Description"=w1730, "Pre-Description"=w1728, "<.?....> Message Code"=w1726) -> ("MHandler Error"=w1725:errorcluster)  [unwired: 4 in, 2 out]
        n1133 = Unbundle By Name(w1718) -> ("PlantID"=w1717:string, "SystemID"=w1716:string)
        n1134 = local write "MHandler"(w1725) -> ()
        n1135 = Bundle("PlantID"=w1717, "SystemID"=w1716) -> (w1715:cluster{"PlantID":string, "SystemID":string})  [unwired: 1 in]
        n1136 = Build Array(w1719) -> (w1720:string[])
        n1137 = call "DB - [CMS].[Execute].[ActiveProcess].vi"("Application"="SRTRS", "[PlantId],[SystemId]"=w1715, "DB - CMS Execute ActiveProcess"=DB_-_CMS_Execute_Active_Process."UPDATE [Execute].[ActiveProcess]", "[Execute].[ActiveProcess]\n2014-10-14 14:58"=w1721, "<Data>"=w1720) -> ("SUMMARY"=w1724:errorcluster)  [unwired: 11 in, 3 out]
        n1138 = local write "DB"(w1724) -> ()
        n1139 = disable-structure shown="Disabled" {
          frame Disabled {
            n1140 = call "DB - [CMS].[Execute].[ActiveProcess].vi"() -> ()  [unwired: 16 in, 4 out]
          }
          frame Enabled {
          }
        }
      }
      event "-------------------------------             Report TAB        ------------------------------------": Value Change {
        n1141 = event-data() -> ()  [unwired: 1 in, 6 out]
      }
      event Mouse Down? {
        n1142 = event-data() -> ("CtlRef"=w1755:refnum<vi>, "Coords"=w1756:T64)  [unwired: 1 in, 6 out]
        n1143 = property on="Property Node" class="CmbBox (strict)"(reference=w1755) -> (reference out=w1757:refnum<vi>, "Text.Left"=w1761:i32, "Text.Width"=w1760:u32)  [unwired: 1 in, 1 out]
        n1144 = Unbundle By Name(w1756) -> ("Horizontal"=w1759:i32)
        n1145 = Add(x=w1761, y=w1760) -> (x+y=w1758:u32)
        n1146 = local read "DB - Report"() -> (w1754:bool)
        n1147 = Greater?(x=w1759, y=w1758) -> (0:w1753:bool)
        n1148 = And(x=w1753, y=w1754) -> (x .and. y?=w1752:bool)
        n1149 = case shown="True" w1752 {
          tunnel: [_ w1762] -> _
          tunnel: w1757 -> [_ w1772]
          frame False {
          }
          frame True {
            w1773 = "%" ("replace string (\"\")")
            # "-- Reinehold Systems Solutions\n-- 2014-10-03\n\nUSE [SRTRS]\nGO\n\nINSERT INTO [Execute].[ReportList]\n           ([TransactionNo]\n           ,[TransactionRunNo]\n           ,[ReportRunNo]\n           ,[OrderNo]\n           ,[PlantId]\n           ,[StationId]\n           ,[AdditionalOrderNo]\n           ,[NoOfOrders]\n           ,[ReportFilePath]\n           ,[ReportFileName]\n           ,[RawDataSourcePath]\n           ,[RawDataSourceFileName]\n           ,[IsManual]\n           ,[CreatedBy]\n           ,[CreatedOn]\n           ,[Inactive])"
            n1150 = property on="Property Node" class="CmbBox (strict)"(reference=w1772) -> (reference out=w1771:refnum<vi>, "Text.Text"=w1776:string, "Label.Text"=w1769:string)  [unwired: 1 in, 1 out]
            n1151 = Search and Replace String(replace all?=TRUE ("replace all? (F)"), input string=w1776, search string="*", replace string=w1773) -> (result string=w1774:string)  [unwired: 4 in, 3 out]
            n1152 = Concatenate Strings(w1774, w1773) -> (w1770:string)
            n1153 = case shown="\"Selection Order No\", Default" w1769 {
              tunnel: [w1788 w1793] -> w1764
              tunnel: w1770 -> [w1789 w1794]
              frame "Selection Order No", Default {
                n1154 = control-ref of="Selection Transaction No"() -> (w1791:refnum<vi>)
                n1155 = property on="Property Node" class="CmbBox (strict)"(reference=w1791, "Value"="") -> ()  [unwired: 1 in, 2 out]
                n1156 = Bundle("OrderNo", w1789) -> (w1788:cluster{string, string})  [unwired: 1 in]
              }
              frame "Selection Transaction No" {
                n1157 = control-ref of="Selection Order No"() -> (w1796:refnum<vi>)
                n1158 = property on="Property Node" class="CmbBox (strict)"(reference=w1796, "Value"="") -> ()  [unwired: 1 in, 2 out]
                n1159 = Bundle("TransactionNo", w1794) -> (w1793:cluster{string, string})  [unwired: 1 in]
              }
            }
            n1160 = disable-structure shown="Disabled" {
              disable-tunnel: [w1778 _] -> w1763
              frame Disabled {
                w1782 = "[CreatedBy] >= '<A>' AND [CreatedBy] <= '<B>'"  # AND <AND_CONDITION>
                # "NOT FOR MOUSE DOWN?"
                n1161 = property on="Date End" class="AbsTime (strict)"() -> ("Value"=w1780:timestamp)  [unwired: 2 in, 2 out]
                n1162 = property on="Date Start" class="AbsTime (strict)"() -> ("Value"=w1779:timestamp)  [unwired: 2 in, 2 out]
                n1163 = global read "Global SRTRS.vi" "Date Time Format"() -> (w1781:string)
                n1164 = Format Date/Time String(time format string (%c)=w1781, seconds (now)=w1779) -> (date/time string=w1786:string)  [unwired: 1 in]
                n1165 = Format Date/Time String(time format string (%c)=w1781, seconds (now)=w1780) -> (date/time string=w1787:string)  [unwired: 1 in]
                n1166 = Search and Replace String(input string=w1782, search string="<A>", replace string=w1786) -> (result string=w1784:string)  [unwired: 5 in, 3 out]
                n1167 = Search and Replace String(input string=w1784, search string="<B>", replace string=w1787) -> (result string=w1778:string)  [unwired: 5 in, 3 out]
              }
              frame Enabled {
              }
            }
            n1168 = call "DB - [Execute].[ReportList].vi"(2:DB_-_Execute_ReportList_Enum."SELECT [TransactionNo] OR [OrderNo]", "AND <AND_CONDITION>"=w1763, "Search Cluster"=w1764) -> ("data"=w1767:string[][], "SUMMARY"=w1762:errorcluster)  [unwired: 9 in, 2 out]
            n1169 = Index Array(array=w1767, index (col)=0 ("disabled index (col)")) -> (element=w1765:string[])  [unwired: 1 in]
            n1170 = property on="Property Node" class="CmbBox (strict)"(reference=w1771, "Strings[]"=w1765) -> ()  [unwired: 1 in, 2 out]
            n1171 = local write "DB"(w1762) -> ()
          }
        }
        n1172 = event-data() -> ()  [unwired: 2 in, 1 out]
      }
      event "Report Selection.Report Execute Search": Value Change {
        n1173 = event-data() -> ()  [unwired: 1 in, 6 out]
        n1174 = Unbundle By Name("Report Selection") -> ("Date Start"=w1805:timestamp, "Date End"=w1804:timestamp, "Selection Transaction No"=w1802:T5, "Selection Order No"=w1803:T5)
        n1175 = local read "DB - Report"() -> (w1800:bool)
        n1176 = call "Queue - EnQueue to MessageQ.vi"("<NoD> Don't Display to UI"=TRUE, "Message"="{Report Search Execute} User Clicked. " ("string")) -> ()  [unwired: 9 in, 1 out]
        n1177 = call "String - Get Dates.vi"("End Date"=w1804, "Start Date"=w1805) -> ("List of Dates YYYYmmDD"=w1801:string[])  [unwired: 8 in, 1 out]
        n1178 = case shown="True" w1800 {
          tunnel: w1803 -> [w1825 w1887]
          tunnel: w1802 -> [w1824 w1889]
          tunnel: w1801 -> [w1823 _]
          frame False {
            # "Hint: Key in 009.* if you want to search 009xxxxxxxxx\nThis searching format is different from Windows File searching"
            # "<Transaction No>_<Order No>_<Date>_<Time>"
            # "Set Scrollbar to top and deselect any selection"
            # "Key in 009.* if you want to search all Reports that start with 009\nRefer to the PCRE Web site at www.pcre.org for more information about Perl Compatible Regular Expressions."
            n1179 = local read "Reports"() -> (w1812:path)
            n1180 = Empty String/Path?(string/path=w1824) -> (empty?=w1826:bool)
            n1181 = case shown="False" w1826 {
              tunnel: w1825 -> [_ w1862]
              tunnel: w1824 -> [w1859 _]
              tunnel: [w1857 w1860] -> w1822
              frame False {
                # "Skip Selection No"
                # "Use Transaction No."
                n1182 = property on="Selection Order No" class="CmbBox (strict)"("Value"="") -> ()  [unwired: 2 in, 2 out]
                n1183 = Concatenate Strings(w1859, "_", ".*_" ("string")) -> (w1857:string)
              }
              frame True {
                # "Skip Transction No"
